vi "buildADAMrequest.vi"(9 "Aspect":string(combo), 11 "MFCs":T1[](array[typedef])) -> (3 "ADAMrequests":cluster{"String":string, "Setpoint":dbl}[](array[cluster]))   [LabVIEW 2016]
uses:
  MFCdescription.ctl
  MFCcapability.ctl
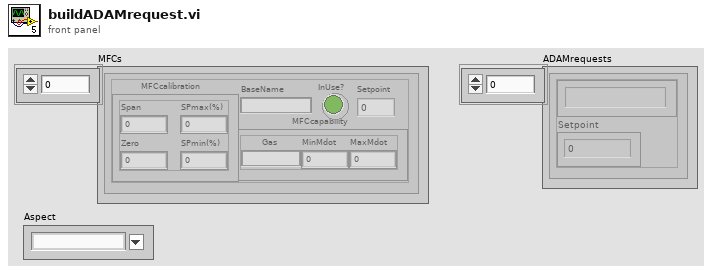
[diagram p1: front panel]
types:
  T1 = typedef "MFCdescription.ctl" = cluster{"BaseName":string, "MFCcalibration":cluster{"Span":dbl, "Zero":dbl, "SPmin(%)":dbl, "SPmax(%)":dbl}, "MFCcapability":T2, "InUse?":bool, "Setpoint":dbl}
  T2 = typedef "MFCcapability.ctl" = cluster{"Gas":string, "MinMdot":dbl, "MaxMdot":dbl}
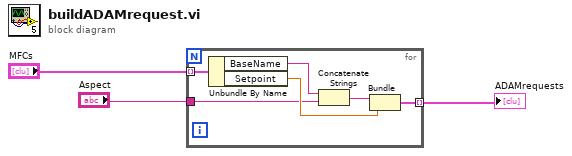
[diagram p0: block diagram]
diagram:
  n1 = for {
    tunnel: "MFCs" -> [w9] mode=indexing
    tunnel: [w7] -> w3 mode=indexing
    tunnel: "Aspect" -> [w4]
    n2 = Unbundle By Name(w9) -> ("BaseName"=w6:string, "Setpoint"=w5:dbl)
    n3 = Concatenate Strings(w6, w4) -> (w8:string)
    n4 = Bundle(w8, "Setpoint"=w5) -> (w7:cluster{string, "Setpoint":dbl})  [unwired: 1 in]
  }
  "ADAMrequests" <- w3
